vi "test2.vi"() -> ()   [LabVIEW 2020]
doc: "Trial"
panel:
  out "x+y":dbl
  in  "y":dbl
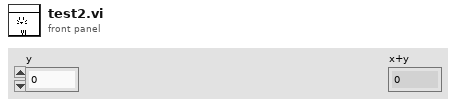
[diagram p1: front panel]
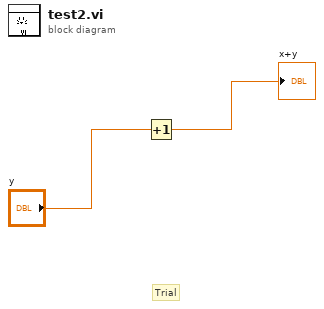
[diagram p0: block diagram]
diagram:
  # "Trial"
  n1 = Increment(x="y") -> (x+1=→"x+y":dbl)
